vi "DMSV.get_node_data.vi"(0 "nodeNotifiers":refnum<notifier>[][](array[refnum]), 5 "error in (no error)":errorcluster) -> (14 "nodeNotifiers (out)":refnum<notifier>[][](array[refnum]), 15 "CPU":sgl[](array[numeric]), 16 "Mem":i32[](array[numeric]), 17 "OS":string[](array[string]), 18 "link?":bool[](array[boolean]), 19 "error out":errorcluster)   [LabVIEW 2014, in "DMSViewer.lvlib"]
doc: "Gets the DIM data of nodes.\n\nauthor: Dietrich Beck, GSI\n\nLicense Agreement for this software:\n\nCopyright (C)\nGesellschaft für Schwerionenforschung, GSI\nPlanckstr. 1\n64291 Darmstadt\nGermany\n\nContact: D.Beck@gsi.de \n\nThis program is free software; you can redistribute it and/or modify it under the terms of the GNU General Public License as published by the Free Software Foundation; either version 2 of the license, or (at your option) any later version.\n\nThis program is distributed in the hope that it will be useful, but WITHOUT ANY WARRANTY; without even the implied warranty of MERCHANTABILITY or FITNESS FOR A PARTICULAR PURPOSE. See the GNU General License for more details (http://www.gnu.org).\n\nGesellschaft für Schwerionenforschung, GSI\nPlanckstr. 1, 64291 Darmstadt, Germany\nFor all questions and ideas contact: M.Richter@gsi.de, H.Brand@gsi.de or D.Beck@gsi.de.\nLast update: 10-OCT-2004"
uses:
  DMSViewer.lvlib
  CSlibraries-extern/DimLVEvent/LVDimInterface/LVDimInterface.lvlib
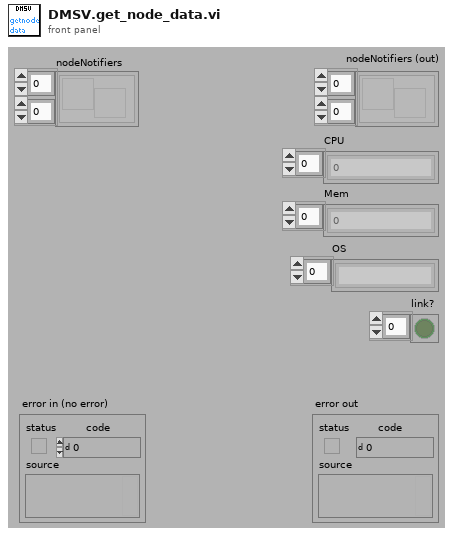
[diagram p1: front panel]
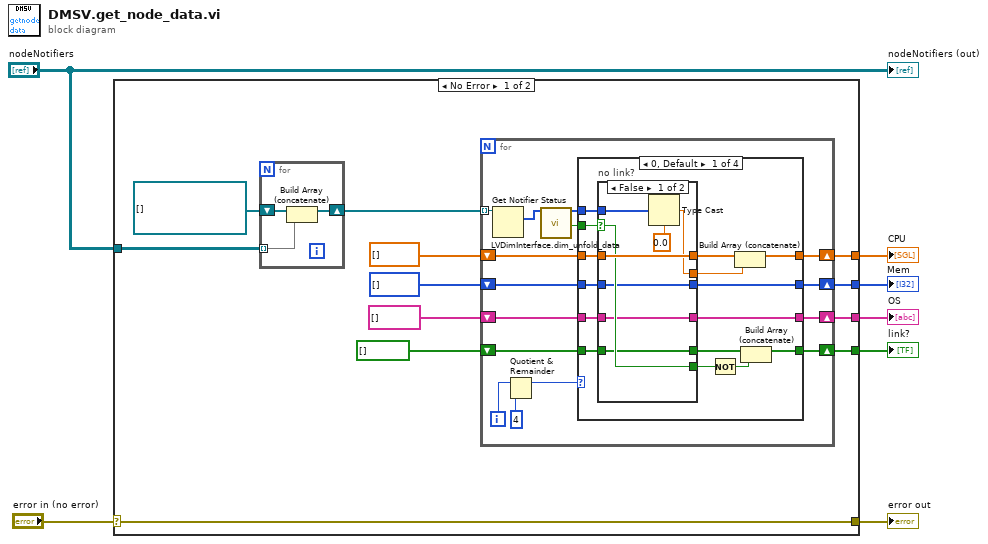
[diagram p0: block diagram]
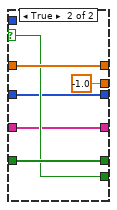
[diagram p2: hidden frame]
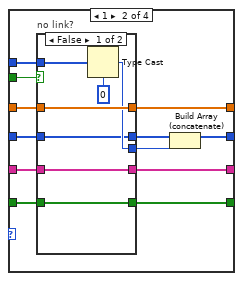
[diagram p3: hidden frame]
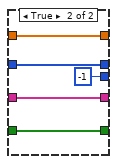
[diagram p4: hidden frame]
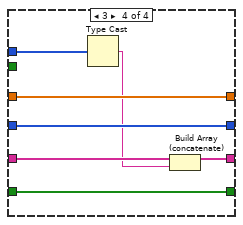
[diagram p7: hidden frame]
diagram:
  n1 = case shown="No Error" "error in (no error)" {
    selector: "error in (no error)" -> [w9 w116]
    tunnel: [w9 w116] -> w6
    tunnel: "nodeNotifiers" -> [w19 _]
    tunnel: [w10 _] -> w1
    tunnel: [w11 _] -> w2
    tunnel: [w12 _] -> w3
    tunnel: [w13 _] -> w4
    frame No Error {
      n2 = for {
        tunnel: w19 -> [w113] mode=indexing
        shift-right: [w115] -> w8
        shift-left: refnum<notifier>[] [] -> [w114]
        n3 = Build Array (concatenate)(w114, w113) -> (w115:refnum<notifier>[])
      }
      n4 = for {
        shift-right: [w28] -> w10
        shift-left: sgl[] [] -> [w29]
        shift-right: [w26] -> w13
        shift-left: bool[] [] -> [w27]
        shift-right: [w24] -> w11
        shift-left: i32[] [] -> [w25]
        shift-right: [w22] -> w12
        shift-left: string[] [] -> [w23]
        tunnel: w8 -> [w21] mode=indexing
        i -> [w34]
        n5 = Get Notifier Status(notifier=w21) -> (current notification=w20:i8[])  [unwired: 1 in, 4 out]
        n6 = Quotient & Remainder(x=w34, y=4) -> (x-y*floor(x/y)=w32:i32)  [unwired: 1 out]
        n7 = call "LVDimInterface.dim_unfold_data.vi"("rawData"=w20) -> ("data"=w31:i8[], "no link"=w30:bool)  [unwired: 15 in, 2 out]
        n8 = case shown="0, Default" w32 {
          tunnel: w31 -> [w49 w74 w96 w112]
          tunnel: w30 -> [w36 w75 w97 _]
          tunnel: w29 -> [w48 w73 w95 w109]
          tunnel: [w45 w68 w91 w109] -> w28
          tunnel: w27 -> [w47 w72 w94 w106]
          tunnel: [w42 w64 w88 w106] -> w26
          tunnel: w25 -> [w40 w71 w93 w111]
          tunnel: [w39 w66 w90 w111] -> w24
          tunnel: w23 -> [w38 w70 w92 w110]
          tunnel: [w37 w69 w89 w107] -> w22
          frame 0, Default {
            n9 = case "no link?" shown="False" w36 {
              selector: w36 -> [w53 w60]
              tunnel: w49 -> [w57 _]
              tunnel: w48 -> [w55 w63]
              tunnel: [w55 w63] -> w46
              tunnel: w47 -> [w52 w61]
              tunnel: [w54 sgl -1.0] -> w44
              tunnel: [w53 w60] -> w41
              tunnel: [w52 w61] -> w43
              tunnel: [w51 w59] -> w39
              tunnel: w40 -> [w51 w59]
              tunnel: [w50 w58] -> w37
              tunnel: w38 -> [w50 w58]
              frame False {
                n10 = Type Cast(type=sgl 0.0, x=w57) -> (*(type *) &x=w54:sgl)
              }
              frame True {
              }
            }
            n11 = Not(x=w41) -> (.not. x?=w35:bool)
            n12 = Build Array (concatenate)(w46, w44) -> (w45:sgl[])
            n13 = Build Array (concatenate)(w43, w35) -> (w42:bool[])
          }
          frame 1 {
            n14 = case "no link?" shown="False" w75 {
              tunnel: w74 -> [w82 _]
              tunnel: w73 -> [w80 w87]
              tunnel: [w80 w87] -> w68
              tunnel: w72 -> [w78 w85]
              tunnel: [w79 -1] -> w65
              tunnel: [w78 w85] -> w64
              tunnel: [w77 w84] -> w67
              tunnel: w71 -> [w77 w84]
              tunnel: [w76 w83] -> w69
              tunnel: w70 -> [w76 w83]
              frame False {
                n15 = Type Cast(type=0, x=w82) -> (*(type *) &x=w79:i32)
              }
              frame True {
              }
            }
            n16 = Build Array (concatenate)(w67, w65) -> (w66:i32[])
          }
          frame 2 {
            n17 = case "no link?" shown="False" w97 {
              tunnel: w96 -> [_ _]
              tunnel: w95 -> [w101 w105]
              tunnel: [w101 w105] -> w91
              tunnel: w94 -> [w100 w104]
              tunnel: [w100 w104] -> w88
              tunnel: [w99 w103] -> w90
              tunnel: w93 -> [w99 w103]
              tunnel: [w98 w102] -> w89
              tunnel: w92 -> [w98 w102]
              frame False {
              }
              frame True {
              }
            }
          }
          frame 3 {
            n18 = Type Cast(x=w112) -> (*(type *) &x=w108:string)  [unwired: 1 in]
            n19 = Build Array (concatenate)(w110, w108) -> (w107:string[])
          }
        }
      }
    }
    frame Error {
    }
  }
  "error out" <- w6
  "link?" <- w4
  "OS" <- w3
  "Mem" <- w2
  "CPU" <- w1
  "nodeNotifiers (out)" <- "nodeNotifiers"
